vi "complex XY.vi"(10 "f":dbl[](array[numeric]), 11 "数组":cdb[](array[numeric])) -> (2 "IM":cluster{"X":dbl, "Y":dbl}[](graph), 3 "RE":cluster{"X":dbl, "Y":dbl}[](graph))   [LabVIEW 2018]
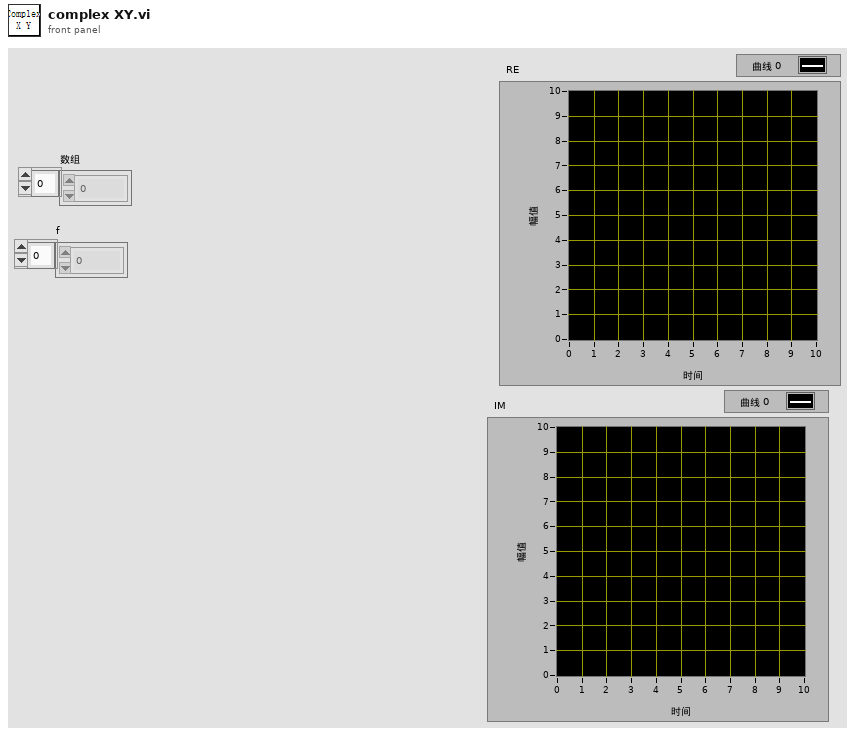
[diagram p1: front panel]
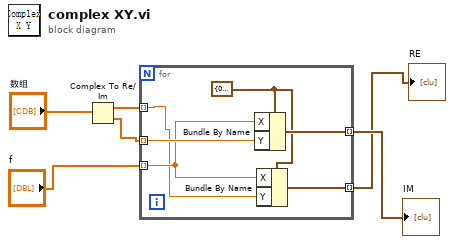
[diagram p0: block diagram]
diagram:
  n1 = Complex To Re/Im(x + iy="数组") -> (x=w6:dbl[], y=w4:dbl[])
  n2 = for {
    tunnel: w6 -> [w8] mode=indexing
    tunnel: w4 -> [w12] mode=indexing
    tunnel: "f" -> [w9] mode=indexing
    tunnel: [w11] -> w2 mode=indexing
    tunnel: [w7] -> w1 mode=indexing
    w10 = cluster{"X":dbl, "Y":dbl} {"X"=0.0, "Y"=0.0}
    n3 = Bundle By Name(cluster=w10, "X"=w9, "Y"=w12) -> (w11:cluster{"X":dbl, "Y":dbl})
    n4 = Bundle By Name(cluster=w10, "X"=w9, "Y"=w8) -> (w7:cluster{"X":dbl, "Y":dbl})
  }
  "RE" <- w1
  "IM" <- w2
